vi "Normalizzazzione Plot.vi"(5 "file path out (dialog if empty)":path, 6 "External File?":bool, 7 "file path (dialog if empty)":path, 11 "Spectrum In":dbl[][](array[numeric])) -> (3 "Spectrum Out":dbl[][](array[numeric]))   [LabVIEW 2023]
uses:
  <vilib>/Utility/file.llb/Read Delimited Spreadsheet (DBL).vi
  <vilib>/Utility/file.llb/Write Delimited Spreadsheet (DBL).vi
panel:
  out "XY Graph 2":cluster{"all rows":dbl[], "all rows":dbl[]}(graph)
  out "XY Graph":cluster{"all rows":dbl[], "all rows":dbl[]}(graph)
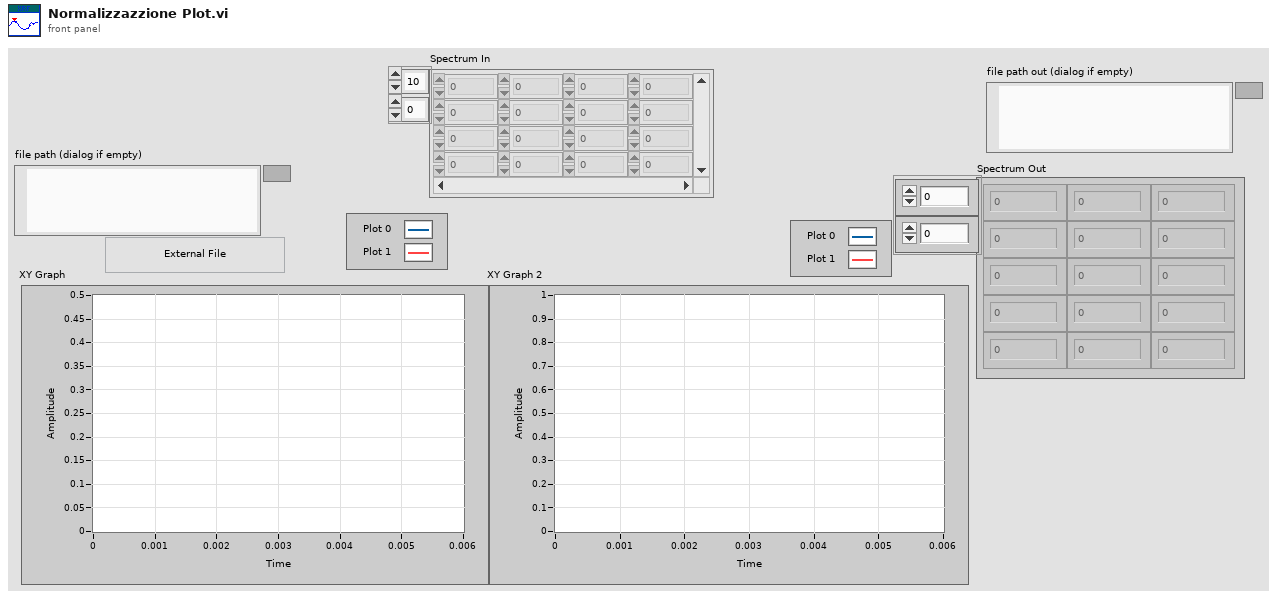
[diagram p1: front panel]
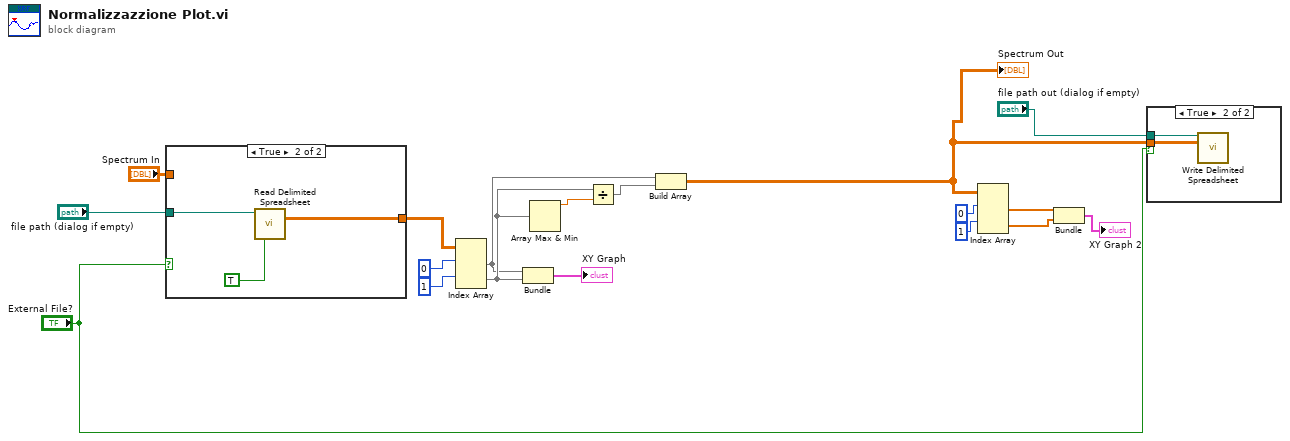
[diagram p0: block diagram]
diagram:
  n1 = case shown="True" "External File?" {
    tunnel: [w19 w21] -> w18
    tunnel: "file path (dialog if empty)" -> [_ w20]
    tunnel: "Spectrum In" -> [w19 _]
    frame False {
    }
    frame True {
      n2 = call-poly <vilib>:"Read Delimited Spreadsheet.vi"("file path (dialog if empty)"=w20, "transpose? (F)"=TRUE) -> ("all rows"=w21:dbl[][])  [unwired: 8 in, 5 out]
    }
  }
  n3 = Index Array(array=w18, index (row) #1=0 ("disabled index (col)"), index (row) #2=1 ("index (col)")) -> (element #1=w8:dbl[], element #2=w10:dbl[])  [unwired: 2 in]
  n4 = Bundle("all rows"=w8, "all rows"=w10) -> (→"XY Graph":cluster{"all rows":dbl[], "all rows":dbl[]})  [unwired: 1 in]
  n5 = Array Max & Min(array=w10) -> (max value=w9:dbl)  [unwired: 3 out]
  n6 = Divide(x=w10, y=w9) -> (x/y=w7:dbl[])
  n7 = Build Array(w8, w7) -> (w6:dbl[][])
  "Spectrum Out" <- w6
  n8 = Index Array(array=w6, index (row) #1=0 ("disabled index (col)"), index (row) #2=1 ("index (col)")) -> (element #1=w17:dbl[], element #2=w16:dbl[])  [unwired: 2 in]
  n9 = Bundle(w17, w16) -> (→"XY Graph 2":cluster{dbl[], dbl[]})  [unwired: 1 in]
  n10 = case shown="True" "External File?" {
    tunnel: w6 -> [_ w24]
    tunnel: "file path out (dialog if empty)" -> [_ w23]
    frame False {
    }
    frame True {
      n11 = call-poly <vilib>:"Write Delimited Spreadsheet.vi"("file path (dialog if empty)"=w23, "2D data"=w24) -> ()  [unwired: 12 in, 2 out]
    }
  }
